vi "VPI Open Device.vi"(9 "Reserved":i32, 10 "DevIndex":i32, 11 "DevType":i32) -> (3 "function return":i32)   [LabVIEW 2010, in "ControlPWM.lvlib"]
doc: "int WINAPI VPI_OpenDevice(int DevType,int DevIndex,int Reserved);"
uses:
  ControlPWM.lvlib
  ControlPWM/Ginkgo_Driver.dll
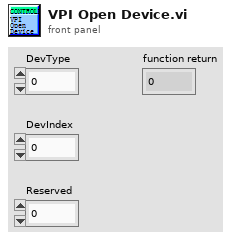
[diagram p1: front panel]
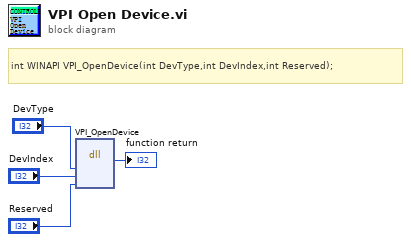
[diagram p0: block diagram]
diagram:
  # "int WINAPI VPI_OpenDevice(int DevType,int DevIndex,int Reserved);"
  n1 = dll-call lib="E:/Project/vt_ginkgo/truck/Ginkgo Driver/vs2010/Ginkgo_USB-I2C&SPI&CAN_API_v2.0.3.3/lib/labview_32bit/ControlPWM/Ginkgo_Driver.*" fn="VPI_OpenDevice"("DevType"="DevType", "DevIndex"="DevIndex", "Reserved"="Reserved") -> (→"function return":i32)  [unwired: 6 in, 2 out]
